vi "Get BPG Voltage.vi"(8 "error in (no error)":errorcluster, 10 "BPG Voltage":waveform(dbl)[](array[waveform]), 11 "BPG in":refnum<class "BPG.lvclass">) -> (0 "error out":errorcluster, 3 "BPG out":refnum<class "BPG.lvclass">)   [LabVIEW 2021, in "BPG.lvlib" / "BPG.lvclass"]
uses:
  BPG.lvclass
  <vilib>/ActorFramework/Actor/Actor.lvclass
  BPG Pressure/BPG Pressure Messages/BPG Pressure Msg/BPG Pressure Msg.lvclass
  Color-Level-Comparison/Colors.ctl
  <userlib>/_MGI/1D Array/MGI Average/MGI Average (DBL[]).vi
  C:/Program Files/National Instruments/LabVIEW 2021/vi.lib/ActorFramework/Actor/Actor.lvclass
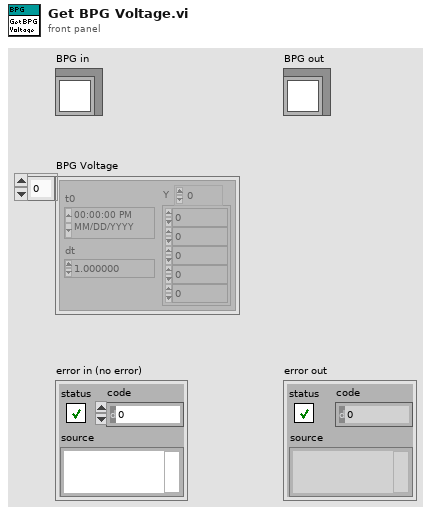
[diagram p1: front panel]
types:
  T1 = typedef "Colors.ctl" = cluster{"Green":u32, "Yellow":u32, "Red":u32}
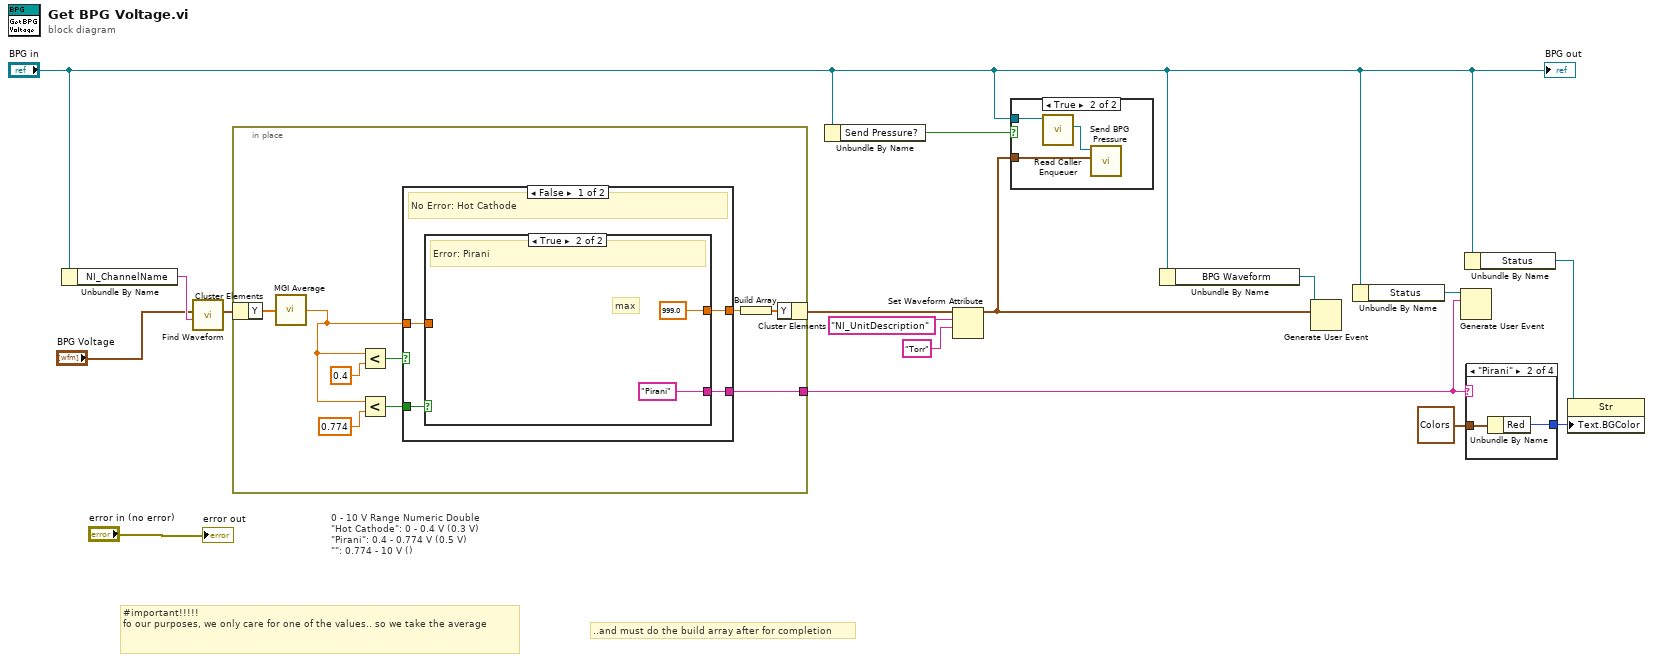
[diagram p0: block diagram]
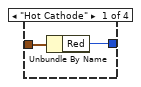
[diagram p3: hidden frame]
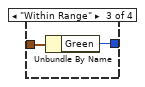
[diagram p4: hidden frame]
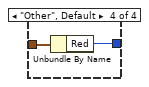
[diagram p5: hidden frame]
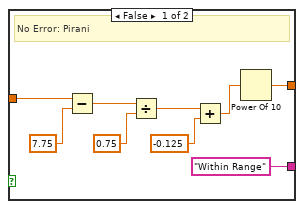
[diagram p6: hidden frame]
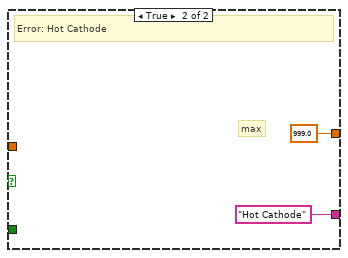
[diagram p7: hidden frame]
diagram:
  # "..and must do the build array after for completion"
  # "#important!!!!!\nfo our purposes, we only care for one of the values.. so we take the average"
  # "0 - 10 V Range Numeric Double\n\"Hot Cathode\": 0 - 0.4 V (0.3 V)\n\"Pirani\": 0.4 - 0.774 V (0.5 V)\n\"\": 0.774 - 10 V ()"
  n1 = Unbundle By Name("BPG in") -> ("NI_ChannelName"=w9:string)
  n2 = call "Find Waveform.vi"("NI_ChannelName"=w9, "Waveform"="BPG Voltage") -> ("Last Waveform"=w10:waveform(dbl))  [unwired: 8 in, 1 out]
  n3 = in-place {
    in-place-border: [w25] -> w12
    n4 = in-place-cluster #1(w10) -> ("Y"=w18:dbl[])
    n5 = call-poly <userlib>:"MGI Average.vi"("Double[]"=w18) -> ("Average"=w17:dbl)  [unwired: 1 in]
    n6 = Less?(x=w17, y=0.4) -> (x < y?=w22:bool)
    n7 = Less?(x=w17, y=0.774) -> (x < y?=w23:bool)
    n8 = case shown="False" w22 {
      tunnel: w23 -> [w29 _]
      tunnel: [w28 999.0] -> w24
      tunnel: w17 -> [w27 _]
      tunnel: [w26 "Hot Cathode"] -> w25
      frame False {
        # "No Error: Hot Cathode"
        n9 = case shown="True" w29 {
          tunnel: [w38 999.0] -> w28
          tunnel: w27 -> [w37 _]
          tunnel: ["Within Range" "Pirani"] -> w26
          frame False {
            # "No Error: Pirani"
            n10 = Subtract(x=w37, y=7.75) -> (x-y=w35:dbl)
            n11 = Divide(x=w35, y=0.75) -> (x/y=w33:dbl)
            n12 = Add(x=w33, y=-0.125) -> (x+y=w31:dbl)
            n13 = Power Of 10(x=w31) -> (10^x=w38:dbl)
          }
          frame True {
            # "max"
            # "Error: Pirani"
          }
        }
      }
      frame True {
        # "max"
        # "Error: Hot Cathode"
      }
    }
    n14 = Build Array(w24) -> (w19:dbl[])
    n15 = in-place-cluster #1("Y"=w19) -> (w2:waveform(dbl))
  }
  n16 = Unbundle By Name("BPG in") -> ("Send Pressure?"=w8:bool)
  n17 = Set Waveform Attribute(5:"Torr" ("name"), 6:"NI_UnitDescription" ("name"), 7:w2) -> (3:w1:waveform(dbl))  [unwired: 1 in, 2 out]
  n18 = case shown="True" w8 {
    tunnel: "BPG in" -> [_ w45]
    tunnel: w1 -> [_ w43]
    frame False {
    }
    frame True {
      n19 = call <vilib>:"Read Caller Enqueuer.vi"("Actor"=w45) -> ("Caller Enqueuer"=w44:refnum<class "Message Enqueuer.lvclass">)  [unwired: 10 in]
      n20 = call "Send BPG Pressure.vi"("BPG Pressure"=w43, "Message Enqueuer"=w44) -> ()  [unwired: 8 in, 2 out]
    }
  }
  n21 = Unbundle By Name("BPG in") -> ("BPG Waveform"=w15:refnum<user-event>)
  n22 = Generate User Event(user event=w15, event data cluster=w1) -> ()  [unwired: 2 in, 2 out]
  n23 = Unbundle By Name("BPG in") -> ("Status"=w14:refnum<user-event>)
  n24 = Generate User Event(user event=w14, event data cluster=w12) -> ()  [unwired: 2 in, 2 out]
  n25 = Unbundle By Name("BPG in") -> ("Status"=w13:refnum<vi>)
  n26 = case shown="\"Pirani\"" w12 {
    tunnel: [w46 w48 w50 w52] -> w11
    tunnel: T1 {"Green"=65408, "Yellow"=16777088, "Red"=16744576} ("Colors") -> [w47 w49 w51 w53]
    frame "Hot Cathode" {
      n27 = Unbundle By Name(w47) -> ("Red"=w46:u32)
    }
    frame "Pirani" {
      n28 = Unbundle By Name(w49) -> ("Red"=w48:u32)
    }
    frame "Within Range" {
      n29 = Unbundle By Name(w51) -> ("Green"=w50:u32)
    }
    frame "Other", Default {
      n30 = Unbundle By Name(w53) -> ("Red"=w52:u32)
    }
  }
  n31 = property class="Str"(reference=w13, "Text.BGColor"=w11) -> ()  [unwired: 1 in, 2 out]
  "error out" <- "error in (no error)"
  "BPG out" <- "BPG in"
